vi "Write Configeration Data.vi"(8 "error in":errorcluster, 9 "Volt Channel":T1={"Index"=[], "Chl Name"=[], "Scale"=[], "Offset"=[], "Sample Rate"=100, "Device Name"="", "Channel"=""}, 10 "File Refnum":variant, 11 "CSV File in":refnum<class "CSV File.lvclass">) -> (0 "error out":errorcluster, 3 "CSV File out":refnum<class "CSV File.lvclass">)   [LabVIEW 2021, in "CSV File.lvclass"]
doc: "This vi helps to write Sample Rate, Channel Index, Channel Name, Scale and Offset into a CSV file."
uses:
  CSV File.lvclass
  Control/Volt Chl.ctl
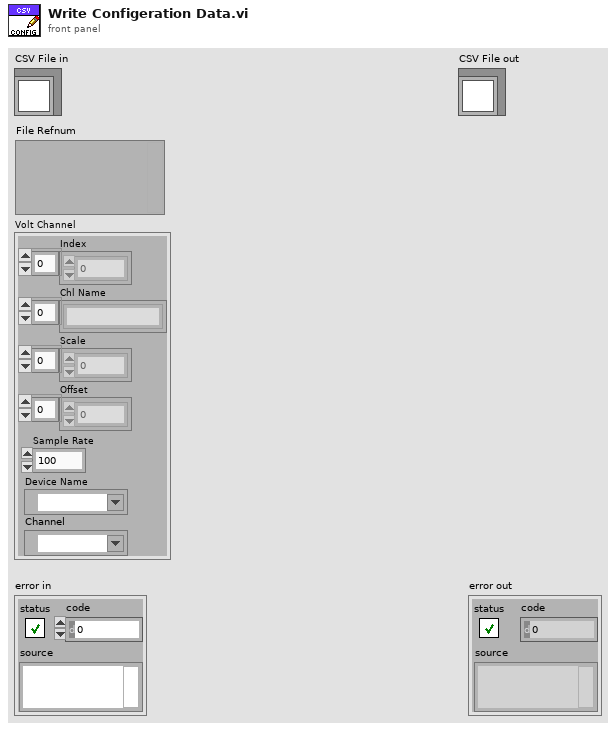
[diagram p1: front panel]
types:
  T1 = typedef "Volt Chl.ctl" = cluster{"Index":i32[], "Chl Name":string[], "Scale":dbl[], "Offset":dbl[], "Sample Rate":i32, "Device Name":tag, "Channel":tag}
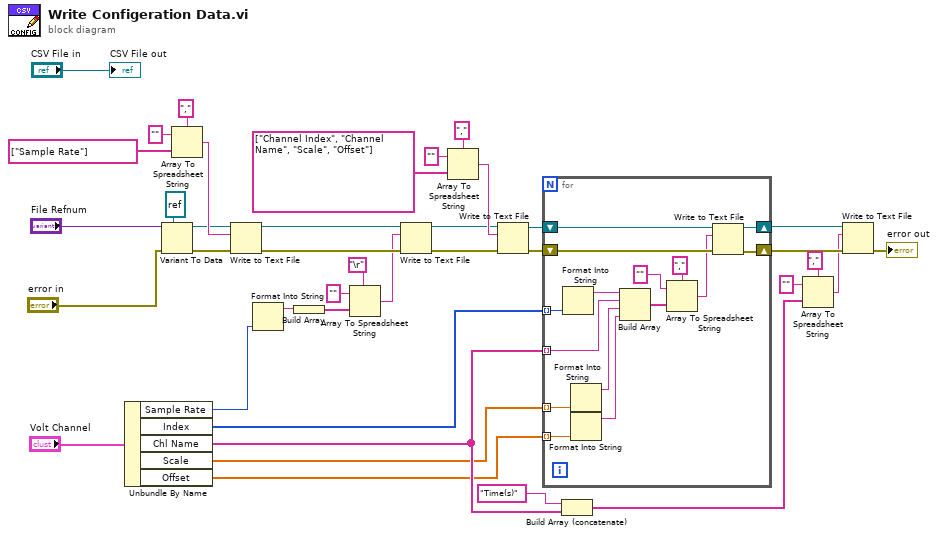
[diagram p0: block diagram]
diagram:
  n1 = Unbundle By Name("Volt Channel") -> ("Sample Rate"=w13:i32, "Index"=w25:i32[], "Chl Name"=w24:string[], "Scale"=w23:dbl[], "Offset"=w22:dbl[])
  n2 = Variant To Data(error in="error in", type=refnum<file> refnum ("CSV Refnum"), Variant="File Refnum") -> (data=w6:refnum<file>, error out=w5:errorcluster)
  n3 = Array To Spreadsheet String(delimiter (Tab)=",", array=string[] ["Sample Rate"], 3:"" ("format string")) -> (spreadsheet string=w15:string)
  n4 = Write to Text File(file (use dialog)=w6, text=w15, error in=w5) -> (refnum out=w21:refnum<file>, error out=w20:errorcluster)  [unwired: 1 in, 1 out]
  n5 = Format Into String(w13) -> (resulting string=w12:string)  [unwired: 3 in, 1 out]
  n6 = Build Array(w12) -> (w9:string[])
  n7 = Array To Spreadsheet String(delimiter (Tab)="\r", array=w9, 3:"" ("format string")) -> (spreadsheet string=w8:string)
  n8 = Write to Text File(file (use dialog)=w21, text=w8, error in=w20) -> (refnum out=w19:refnum<file>, error out=w18:errorcluster)  [unwired: 1 in, 1 out]
  n9 = Array To Spreadsheet String(delimiter (Tab)=",", array=string[] ["Channel Index", "Channel Name", "Scale", "Offset"], 3:"" ("format string")) -> (spreadsheet string=w39:string)
  n10 = Write to Text File(file (use dialog)=w19, text=w39, error in=w18) -> (refnum out=w35:refnum<file>, error out=w36:errorcluster)  [unwired: 1 in, 1 out]
  n11 = for {
    tunnel: w25 -> [w54] mode=indexing
    tunnel: w23 -> [w53] mode=indexing
    tunnel: w22 -> [w52] mode=indexing
    tunnel: w24 -> [w46] mode=indexing
    shift-right: [w48] -> w34
    shift-left: w36 -> [w49]
    shift-right: [w40] -> w33
    shift-left: w35 -> [w41]
    n12 = Format Into String(w54) -> (resulting string=w51:string)  [unwired: 3 in, 1 out]
    n13 = Format Into String(w53) -> (resulting string=w47:string)  [unwired: 3 in, 1 out]
    n14 = Format Into String(w52) -> (resulting string=w50:string)  [unwired: 3 in, 1 out]
    n15 = Build Array(w51, w46, w47, w50) -> (w45:string[])
    n16 = Array To Spreadsheet String(delimiter (Tab)=",", array=w45, 3:"" ("format string")) -> (spreadsheet string=w42:string)
    n17 = Write to Text File(file (use dialog)=w41, text=w42, error in=w49) -> (refnum out=w40:refnum<file>, error out=w48:errorcluster)  [unwired: 1 in, 1 out]
  }
  n18 = Build Array (concatenate)("Time(s)", w24) -> (w29:string[])
  n19 = Array To Spreadsheet String(delimiter (Tab)=",", array=w29, 3:"" ("format string")) -> (spreadsheet string=w31:string)
  n20 = Write to Text File(file (use dialog)=w33, text=w31, error in=w34) -> (error out=→"error out":errorcluster)  [unwired: 1 in, 2 out]
  "CSV File out" <- "CSV File in"
